vi "ReadFlag.vi"(7 "LabVIEW Web Service Request":refnum<class "Web Request.lvclass">, 10 "Room":i32) -> (2 "FlagsState":string)   [LabVIEW 2015]
uses:
  <vilib>/wsapi/Web Request.lvclass
  TypeDef/RoomsActionEnum.ctl
panel:
  # "Use the Web Service Request input terminal to call the VIs on the Web Services palette. Do not remove it from the connector pane unless you don't need access to the palette."
  # "Each additional control wired to the connector pane will be available as an input in the URL. To include an indicator in terminal-mode output (the default setting), it must also be wired to the connector pane."
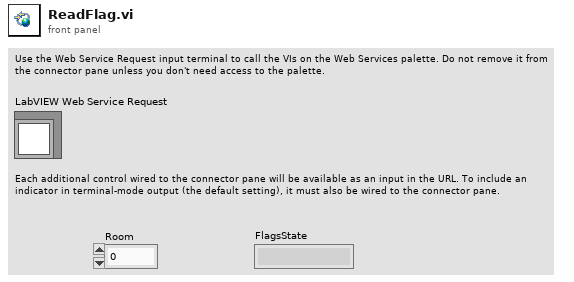
[diagram p1: front panel]
types:
  T1 = typedef "RoomsActionEnum.ctl" = enum16{"Init", "Add Room", "Remove Room", "Read Room", "Read Flag", "Read Flag State", "Write Flag State", "Read Flag Color", "Write Flag Color", "Read Bed Vacant", "Write Bed Vacant", "Read Personnel", "Add Personnel", "Remove Personnel", "Read Requests", "Add Request", "Remove Request", "Read Beacon ID", "Write Beacon ID", "Write Bed URL", "Read Bed URL", "Read Rooms Numbers", "Write Flag"}
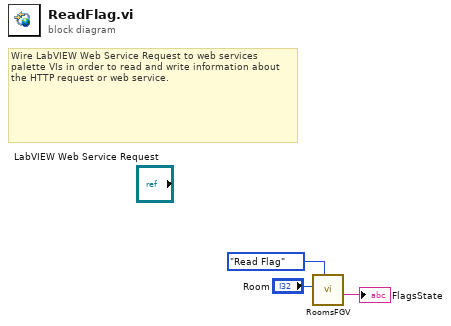
[diagram p0: block diagram]
diagram:
  # "Wire LabVIEW Web Service Request to web services palette VIs in order to read and write information about the HTTP request or web service."
  n1 = call "RoomsFGV.vi"("Actions"=RoomsActionEnum."Read Flag", "Room"="Room") -> ("Data Out"=→"FlagsState":string)  [unwired: 8 in, 1 out]
